vi "ProdaNG.File.Export.TS.vi"(5 "Identification":T1, 6 "reason":string, 7 "TestStepsTree":refnum<vi>, 8 "error in (no error)":errorcluster, 10 "FileContent":T2, 11 "dbHandleIn":i32) -> (0 "error out":errorcluster, 3 "dbHandle":i32)   [LabVIEW 2016]
uses:
  ProdaNG.File.Sequence.ctl
  ProdaNG.Tree.Fglb.Value.ctl
  ProdaNG.File.Step.ctl
  ProdaNG.Tree.Fglb.Action.ctl
  ProdaNG.Tree.Fglb.Data.ctl
  ProdaNG.Tree.Fglb.Element.ctl
  ProdaNG.Configurator.Glb.vi
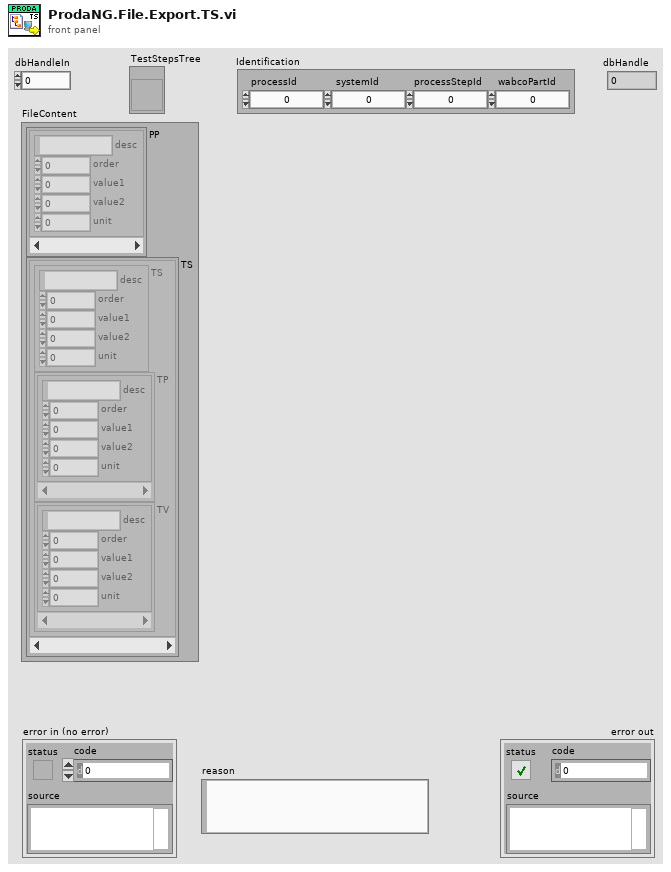
[diagram p1: front panel]
types:
  T1 = cluster{"processId":i32, "systemId":i32, "processStepId":i32, "wabcoPartId":i32}
  T2 = typedef "ProdaNG.File.Sequence.ctl" = cluster{"PP":T3[], "TS":T4[]}
  T3 = typedef "ProdaNG.Tree.Fglb.Value.ctl" = cluster{"desc":string, "order":i32, "value1":dbl, "value2":dbl, "unit":i32}
  T4 = typedef "ProdaNG.File.Step.ctl" = cluster{"TS":T3, "TP":T3[], "TV":T3[]}
  T5 = typedef "ProdaNG.Tree.Fglb.Data.ctl" = cluster{"tag":string, "row":i32, "element":T6, "idx1":i32, "idx2":i32, "file":bool}
  T6 = typedef "ProdaNG.Tree.Fglb.Element.ctl" = enum16{"-", "PP", "TS", "TP", "TV"}
  T7 = typedef "ProdaNG.Tree.Fglb.Action.ctl" = enum16{"init", "add", "get by row", "get by tag", "get by idx"}
  T8 = typedef "ProdaNG.TestStep.ctl" = cluster{"i_id":i32, "processStepId":i32, "testSequence":i32, "testOrder":i32, "mdReason":string, "mdUser":string, "mdTime":string, "description":string}
  T9 = typedef "ProdaNG.TestStepParam.ctl" = cluster{"i_id":i32, "testStepId":i32, "unitId":i32, "contentId":string, "previewId":string, "value":dbl, "valueText":string, "paramSequence":i32, "history":i32, "mdReason":string, "mdUser":string, "mdTime":string, "description":string}
  T10 = typedef "ProdaNG.TestValue.ctl" = cluster{"i_id":i32, "testStepId":i32, "releaseId":i32, "unitId":i32, "contentId":string, "previewId":string, "maximum":dbl, "minimum":dbl, "valueText":string, "testValueSequence":i32, "history":i32, "mdReason":string, "mdUser":string, "mdTime":string, "description":string}
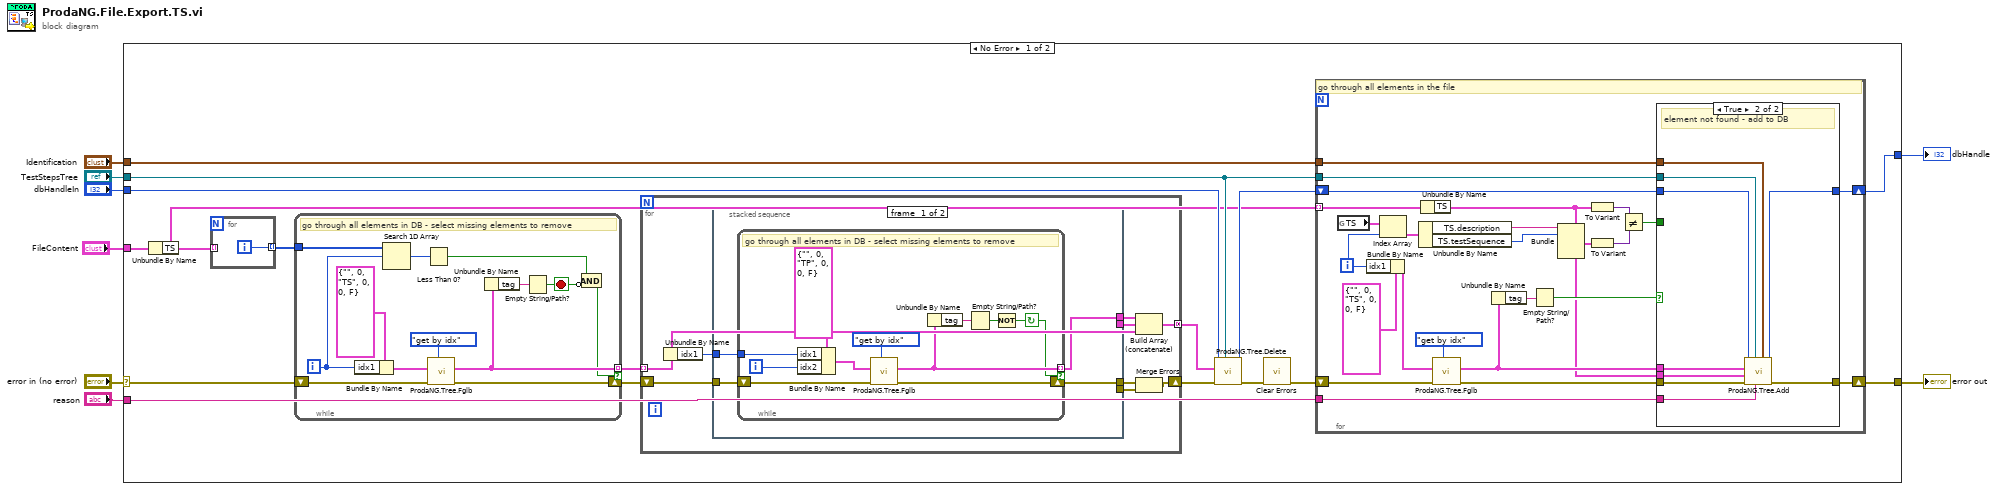
[diagram p0: block diagram]
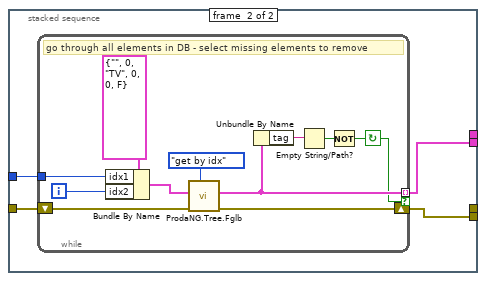
[diagram p2: hidden frame]
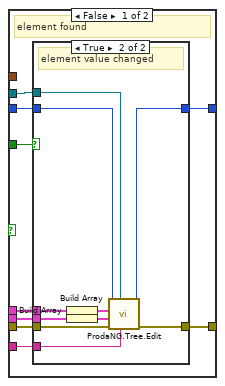
[diagram p3: hidden frame]
diagram:
  n1 = case shown="No Error" "error in (no error)" {
    selector: "error in (no error)" -> [w25 w135]
    tunnel: [w17 w135] -> w8
    tunnel: "dbHandleIn" -> [w23 w134]
    tunnel: [w10 w134] -> w5
    tunnel: "FileContent" -> [w12 _]
    tunnel: "TestStepsTree" -> [w13 _]
    tunnel: "Identification" -> [w15 _]
    tunnel: "reason" -> [w14 _]
    frame No Error {
      n2 = Unbundle By Name(w12) -> ("TS"=w11:T4[])
      n3 = for {
        tunnel: w11 -> [_] mode=indexing
        tunnel: [w65] -> w24 mode=indexing
        i -> [w65]
      }
      n4 = while {
        tunnel: [w74] -> w20 mode=indexing if=w70
        shift-right: [w73] -> w22
        shift-left: w25 -> [w77]
        tunnel: w24 -> [w72]
        i -> [w67]
        stop <- w66 stop-if-true
        # "go through all elements in DB - select missing elements to remove"
        n5 = Bundle By Name(cluster=T5 {"tag"="", "row"=0, "element"=enum."TS", "idx1"=0, "idx2"=0, "file"=FALSE} ("entry in"), "idx1"=w67) -> (w68:T5)
        n6 = Search 1D Array(1D array=w72, element=w67) -> (index of element=w71:i32)  [unwired: 1 in]
        n7 = Less Than 0?(x=w71) -> (x < 0?=w69:bool)
        n8 = call "ProdaNG.Tree.Fglb.vi"("Action (add)"=ProdaNG.Tree.Fglb.Action."get by idx", "error in"=w77, "entry in"=w68) -> ("error out"=w73:errorcluster, "found entry"=w74:T5)  [unwired: 6 in, 1 out]
        n9 = Unbundle By Name(w74) -> ("tag"=w75:string)
        n10 = Empty String/Path?(string/path=w75) -> (empty?=w66:bool)
        n11 = Compound Arithmetic op=AND(w69, invert w66) -> (w70:bool)
      }
      n12 = for {
        tunnel: w20 -> [w30] mode=indexing
        shift-right: [w27] -> w21
        shift-left: w22 -> [w34]
        tunnel: [w26] -> w19 mode=concatenating
        n13 = Unbundle By Name(w30) -> ("idx1"=w32:i32)
        n14 = stacked-sequence {
          tunnel: w34 -> [w38 w53]
          tunnel: [w37 _] -> w33
          tunnel: w32 -> [w36 w52]
          tunnel: [w35 _] -> w29
          tunnel: [_ w51] -> w31
          tunnel: [_ w50] -> w28
          frame #0 {
            n15 = while {
              tunnel: [w45] -> w37 mode=indexing if=w40
              shift-right: [w44] -> w35
              shift-left: w38 -> [w48]
              tunnel: w36 -> [w39]
              i -> [w42]
              stop <- w40 continue-if-true
              # "go through all elements in DB - select missing elements to remove"
              n16 = Bundle By Name(cluster=T5 {"tag"="", "row"=0, "element"=enum."TP", "idx1"=0, "idx2"=0, "file"=FALSE} ("entry in"), "idx1"=w39, "idx2"=w42) -> (w43:T5)
              n17 = call "ProdaNG.Tree.Fglb.vi"("Action (add)"=ProdaNG.Tree.Fglb.Action."get by idx", "error in"=w48, "entry in"=w43) -> ("error out"=w44:errorcluster, "found entry"=w45:T5)  [unwired: 6 in, 1 out]
              n18 = Unbundle By Name(w45) -> ("tag"=w46:string)
              n19 = Empty String/Path?(string/path=w46) -> (empty?=w41:bool)
              n20 = Not(x=w41) -> (.not. x?=w40:bool)
            }
          }
          frame #1 {
            n21 = while {
              tunnel: [w60] -> w51 mode=indexing if=w55
              shift-right: [w59] -> w50
              shift-left: w53 -> [w63]
              tunnel: w52 -> [w54]
              i -> [w57]
              stop <- w55 continue-if-true
              # "go through all elements in DB - select missing elements to remove"
              n22 = Bundle By Name(cluster=T5 {"tag"="", "row"=0, "element"=enum."TV", "idx1"=0, "idx2"=0, "file"=FALSE} ("entry in"), "idx1"=w54, "idx2"=w57) -> (w58:T5)
              n23 = call "ProdaNG.Tree.Fglb.vi"("Action (add)"=ProdaNG.Tree.Fglb.Action."get by idx", "error in"=w63, "entry in"=w58) -> ("error out"=w59:errorcluster, "found entry"=w60:T5)  [unwired: 6 in, 1 out]
              n24 = Unbundle By Name(w60) -> ("tag"=w61:string)
              n25 = Empty String/Path?(string/path=w61) -> (empty?=w56:bool)
              n26 = Not(x=w56) -> (.not. x?=w55:bool)
            }
          }
        }
        n27 = Build Array (concatenate)(w33, w31, w30) -> (w26:T5[])
        n28 = Merge Errors(w29, w28) -> (w27:errorcluster)
      }
      n29 = call "ProdaNG.Tree.Delete.vi"("TestStepsTree"=w13, "error in (no error)"=w21, "Elements to delete"=w19, "dbHandleIn"=w23) -> ("error out"=w18:errorcluster, "dbHandle"=w16:i32)  [unwired: 6 in]
      n30 = call <vilib>:"Clear Errors.vi"("error in (no error)"=w18) -> ("error out"=w9:errorcluster)  [unwired: 5 in, 1 out]
      n31 = for {
        shift-right: [w95] -> w17
        shift-left: w9 -> [w100]
        shift-right: [w92] -> w10
        shift-left: w16 -> [w96]
        tunnel: w11 -> [w87] mode=indexing
        tunnel: w14 -> [w93]
        tunnel: w15 -> [w91]
        tunnel: w13 -> [w90]
        i -> [w80]
        # "go through all elements in the file"
        n32 = global read "ProdaNG.Configurator.Glb.vi" "TS"() -> (w82:cluster{"TS":T8, "TP":T9[], "TV":T10[]}[])
        n33 = Bundle By Name(cluster=T5 {"tag"="", "row"=0, "element"=enum."TS", "idx1"=0, "idx2"=0, "file"=FALSE} ("entry in"), "idx1"=w80) -> (w101:T5)
        n34 = Index Array(array=w82, index=w80) -> (element=w81:cluster{"TS":T8, "TP":T9[], "TV":T10[]})
        n35 = Unbundle By Name(w81) -> ("TS.description"=w89:string, "TS.testSequence"=w83:i32)
        n36 = Unbundle By Name(w87) -> ("TS"=w79:T3)
        n37 = call "ProdaNG.Tree.Fglb.vi"("Action (add)"=ProdaNG.Tree.Fglb.Action."get by idx", "error in"=w100, "entry in"=w101) -> ("error out"=w97:errorcluster, "found entry"=w94:T5)  [unwired: 6 in, 1 out]
        n38 = Unbundle By Name(w94) -> ("tag"=w99:string)
        n39 = Empty String/Path?(string/path=w99) -> (empty?=w98:bool)
        n40 = Bundle(cluster=w79, "desc"=w89, "order"=w83) -> (w88:T3)  [unwired: 3 in]
        n41 = To Variant(anything=w79) -> (Variant=w86:variant)
        n42 = To Variant(anything=w88) -> (Variant=w85:variant)
        n43 = Not Equal?(x=w86, y=w85) -> (x != y?=w84:bool)
        n44 = case shown="True" w98 {
          tunnel: w97 -> [w112 w133]
          tunnel: w96 -> [w108 w132]
          tunnel: [w111 w127] -> w95
          tunnel: w94 -> [w109 w131]
          tunnel: w79 -> [w106 w130]
          tunnel: w93 -> [w110 w129]
          tunnel: [w107 w128] -> w92
          tunnel: w91 -> [_ w126]
          tunnel: w90 -> [w105 w125]
          tunnel: w84 -> [w104 _]
          frame False {
            # "element found"
            n45 = case shown="True" w104 {
              tunnel: w112 -> [w114 w124]
              tunnel: [w114 w123] -> w111
              tunnel: w110 -> [_ w122]
              tunnel: w109 -> [_ w121]
              tunnel: w108 -> [w113 w119]
              tunnel: [w113 w118] -> w107
              tunnel: w106 -> [_ w117]
              tunnel: w105 -> [_ w115]
              frame False {
              }
              frame True {
                # "element value changed"
                n46 = Build Array(w121) -> (w120:T5[])
                n47 = Build Array(w117) -> (w116:T3[])
                n48 = call "ProdaNG.Tree.Edit.vi"("reason"=w122, "TestStepsTree"=w115, "error in (no error)"=w124, "Selected elements values"=w116, "Selected elements"=w120, "dbHandleIn"=w119) -> ("error out"=w123:errorcluster, "dbHandle"=w118:i32)  [unwired: 4 in]
              }
            }
          }
          frame True {
            # "element not found - add to DB"
            n49 = call "ProdaNG.Tree.Add.vi"("Identification"=w126, "reason"=w129, "TestStepsTree"=w125, "error in (no error)"=w133, "Element values"=w130, "Element to add"=w131, "dbHandleIn"=w132) -> ("error out"=w127:errorcluster, "dbHandle"=w128:i32)  [unwired: 3 in]
          }
        }
      }
    }
    frame Error {
    }
  }
  "error out" <- w8
  "dbHandle" <- w5
